vi "DI Scope Data.vi"() -> ()   [LabVIEW 2016]
panel:
  in  "DI Scope Data":sgl[][](array[numeric])
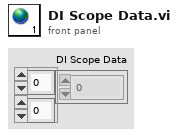
[diagram p1: front panel]
diagram:
